vi "Add Braces.vi"   [LabVIEW 2016, in "Transport.lvclass"]
uses:
  Transport.lvclass
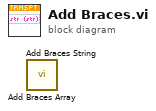
[diagram p0: block diagram]
diagram:
  n1 = call "Add Braces Array.vi"() -> ()  [unwired: 1 in, 1 out]
  n2 = call "Add Braces String.vi"() -> ()  [unwired: 1 in, 1 out]
